vi "Jannson-LVtoJSON.vi"() -> ()   [LabVIEW 2014]
uses:
  ftw-dataflow/ftw/src/core/json/FTW-JSON.lvclass
panel:
  in  "columns":string[](array[string])
  in  "error in":errorcluster
  in  "data":string[][](array[string])
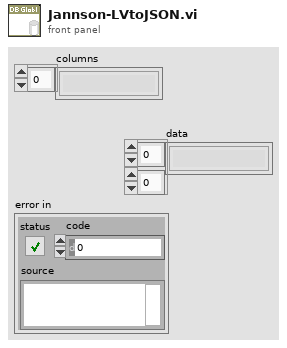
[diagram p1: front panel]
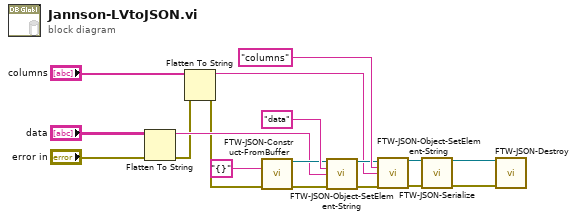
[diagram p0: block diagram]
diagram:
  n1 = Flatten To String(anything="data", error in (no error)="error in") -> (data string=w8:string, error out=w6:errorcluster)  [unwired: 2 in, 1 out]
  n2 = Flatten To String(anything="columns", error in (no error)=w6) -> (data string=w3:string, error out=w4:errorcluster)  [unwired: 2 in, 1 out]
  n3 = call "FTW-JSON-Construct-FromBuffer.vi"("JSON String (UTF-8)"="{}" ("FTW Actor Instance Configuration 2"), "error in"=w4) -> ("JSON Object"=w10:refnum<class "FTW-JSON.lvclass">, "error out"=w11:errorcluster)  [unwired: 12 in]
  n4 = call "FTW-JSON-Object-SetElement-String.vi"("JSON Object"=w10, "Key"="data", "Value"=w8, "error in"=w11) -> ("JSON Object out"=w14:refnum<class "FTW-JSON.lvclass">, "error out"=w15:errorcluster)  [unwired: 10 in]
  n5 = call "FTW-JSON-Object-SetElement-String.vi"("JSON Object"=w14, "Key"="columns", "Value"=w3, "error in"=w15) -> ("JSON Object out"=w2:refnum<class "FTW-JSON.lvclass">, "error out"=w1:errorcluster)  [unwired: 10 in]
  n6 = call "FTW-JSON-Serialize.vi"("JSON Object"=w2, "error in"=w1) -> ("JSON Object out"=w18:refnum<class "FTW-JSON.lvclass">, "error out"=w17:errorcluster)  [unwired: 11 in, 1 out]
  n7 = call "FTW-JSON-Destroy.vi"("JSON Object"=w18, "error in"=w17) -> ()  [unwired: 13 in, 1 out]
